vi "Validate Enum Strings.vi"(8 "error in":errorcluster, 11 "measurement plugin service in":refnum<class "Measurement Plugin Service.lvclass">) -> (0 "error out":errorcluster, 3 "measurement plugin service out":refnum<class "Measurement Plugin Service.lvclass">)   [LabVIEW 2021, in "NI Measurement Plug-In SDK.lvlib"]
uses:
  NI Measurement Plug-In SDK.lvlib
  Measurement Plugin Service/Measurement Plugin Service.lvclass
  Error Strings Global Internal.vi
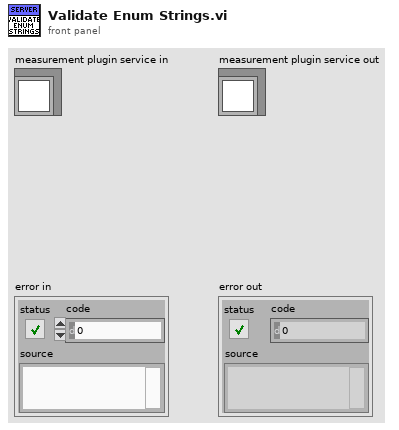
[diagram p1: front panel]
types:
  T1 = typedef "NI Measurement Plug-In SDK.lvlib/Measurement Plugin Service.lvclass/Plugin Paths.ctl" = cluster{"get service descriptor VI path":path, "get type specializations VI path":path, "get UI details VI path":path, "measurement logic VI path":path, "measurement configuration ctl path":path, "measurement results ctl path":path}
  T2 = cluster{"Enum reference out":refnum<vi>, "Label.Text":string}[]
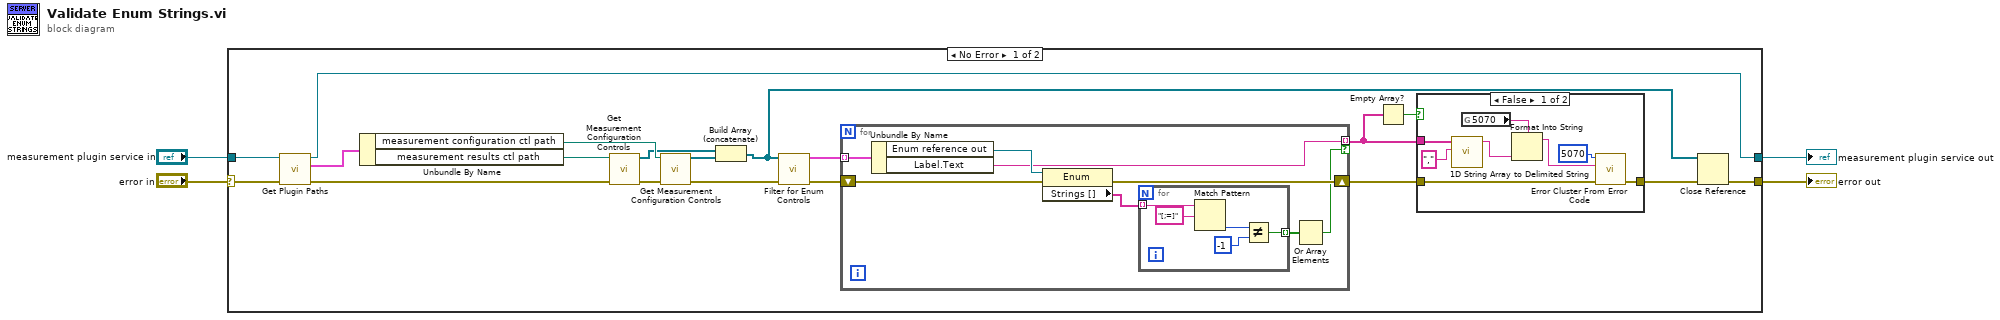
[diagram p0: block diagram]
diagram:
  n1 = case shown="No Error" "error in" {
    selector: "error in" -> [w22 w47]
    tunnel: "measurement plugin service in" -> [w23 w46]
    tunnel: [w7 w47] -> w2
    tunnel: [w11 w46] -> w1
    frame No Error {
      n2 = call-dynamic "Get Plugin Paths.vi"("error in"=w22, "measurement plugin service in"=w23) -> ("error out"=w21:errorcluster, "plugin paths"=w20:T1, "measurement plugin service out"=w11:refnum<class "Measurement Plugin Service.lvclass">)  [unwired: 7 in]
      n3 = Unbundle By Name(w20) -> ("measurement configuration ctl path"=w17:path, "measurement results ctl path"=w18:path)
      n4 = call "Get Measurement Configuration Controls.vi"("error in"=w21, "measurement configuration control path"=w18) -> ("error out"=w19:errorcluster, "controls"=w14:refnum<vi>[])  [unwired: 7 in]
      n5 = call "Get Measurement Configuration Controls.vi"("error in"=w19, "measurement configuration control path"=w17) -> ("error out"=w16:errorcluster, "controls"=w15:refnum<vi>[])  [unwired: 7 in]
      n6 = Build Array (concatenate)(w14, w15) -> (w6:refnum<vi>[])
      n7 = call "Filter for Enum Controls.vi"("error in"=w16, "controls"=w6) -> ("error out"=w12:errorcluster, "enum controls and labels"=w13:T2)  [unwired: 8 in]
      n8 = for {
        tunnel: w13 -> [w31] mode=indexing
        shift-right: [w30] -> w9
        shift-left: w12 -> [w28]
        tunnel: [w26] -> w5 mode=indexing if=w24
        n9 = Unbundle By Name(w31) -> ("Enum reference out"=w29:refnum<vi>, "Label.Text"=w26:string)
        n10 = property class="Enum"(reference=w29, error in=w28) -> (error out=w30:errorcluster, "Strings []"=w27:string[])  [unwired: 1 out]
        n11 = for {
          tunnel: w27 -> [w35] mode=indexing
          tunnel: [w32] -> w25 mode=indexing
          n12 = Match Pattern(string=w35, regular expression="[;=]" ("string")) -> (offset past match=w34:i32)  [unwired: 1 in, 3 out]
          n13 = Not Equal?(x=w34, y=-1) -> (x != y?=w32:bool)
        }
        n14 = Or Array Elements(Boolean array=w25) -> (logical OR=w24:bool)
      }
      n15 = Empty Array?(array=w5) -> (empty?=w10:bool)
      n16 = case shown="False" w10 {
        tunnel: w9 -> [w40 w45]
        tunnel: [w41 w45] -> w8
        tunnel: w5 -> [w39 _]
        frame False {
          n17 = call <vilib>:"1D String Array to Delimited String.vi"("delimiter"=",", "string array"=w39) -> ("delimited string"=w38:string)  [unwired: 9 in]
          n18 = global read "Error Strings Global Internal.vi" "5070"() -> (w42:string)
          n19 = Format Into String(format string=w42, w38) -> (resulting string=w43:string)  [unwired: 2 in, 1 out]
          n20 = call <vilib>:"Error Cluster From Error Code.vi"("error in (no error)"=w40, "error message (\"\")"=w43, "error code (0)"=5070) -> ("error out"=w41:errorcluster)  [unwired: 6 in]
        }
        frame True {
        }
      }
      n21 = Close Reference(reference=w6, error in (no error)=w8) -> (error out=w7:errorcluster)
    }
    frame Error {
    }
  }
  "measurement plugin service out" <- w1
  "error out" <- w2
